vi "sort channels.vi"(7 "Type":T3=enum."Input Register", 8 "error in (no error)":errorcluster, 9 "Starting Index":i32, 10 "Group Name":string, 11 "Item Ref in":T1 format="%.0x") -> (0 "error out":errorcluster, 1 "Next Index":i32, 2 "Inputs":T2[](array[typedef]), 3 "Parent Ref out":T1 format="%.0x", 4 "Refs":T1[](array[typedef]) format="%.0x", 5 "Outputs":T2[](array[typedef]))   [LabVIEW 2015]
uses:
  <vilib>/NI Veristand/Custom Device API/Custom Device API.lvlib
  Modbus Type.ctl
  Shared/Modbus Master Shared.lvlib
  Shared/Controls/Data Model/Channel.ctl
  Modbus Master System Explorer.lvlib
  Shared/Constants.vi
  Shared/Controls/Data Model/DataType.ctl
  Shared/Controls/Data Model/Mapping.ctl
  <vilib>/NI Veristand/Custom Device API/Get Item Property (I32).vi
  <vilib>/NI Veristand/Custom Device API/Custom Device Item Ref.ctl
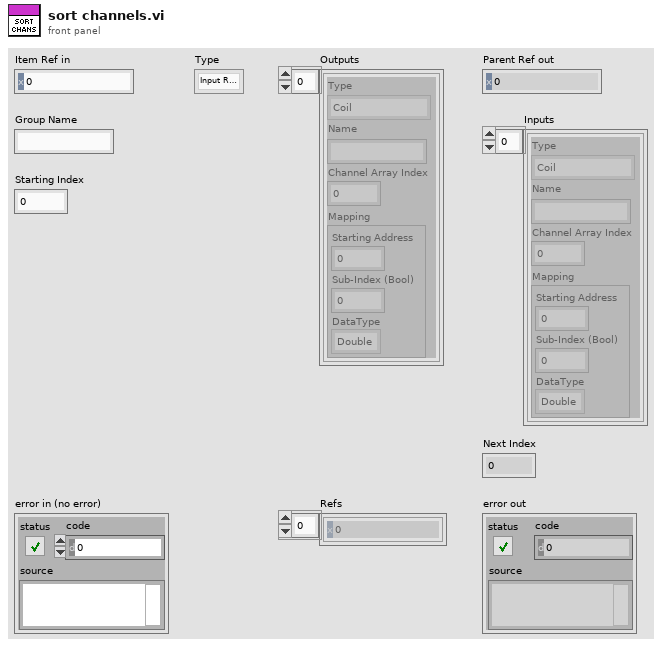
[diagram p1: front panel]
types:
  T1 = typedef "Custom Device API.lvlib/Custom Device Item Ref.ctl" = u64
  T2 = typedef "Modbus Master Shared.lvlib/Channel.ctl" = cluster{"Type":T3, "Name":string, "Channel Array Index":i32, "Mapping":T4}
  T3 = typedef "Modbus Master Shared.lvlib/Modbus Type.ctl" = enum16{"Coil", "Discrete Input", "Holding Register", "Input Register"}
  T4 = typedef "Modbus Master Shared.lvlib/Mapping.ctl" = cluster{"Starting Address":u16, "Sub-Index (Bool)":u16, "DataType":T5}
  T5 = typedef "Modbus Master Shared.lvlib/DataType.ctl" = enum16{"Double", "Single", "I64", "I32", "I16", "I8", "U64", "U32", "U16", "U8", "Boolean", "String"}
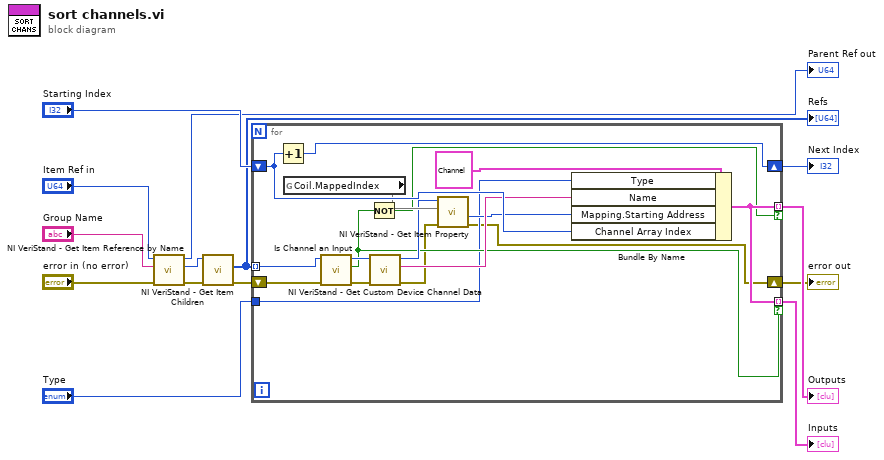
[diagram p0: block diagram]
diagram:
  n1 = call <vilib>:"NI VeriStand - Get Item Reference by Name.vi"("error in (no error)"="error in (no error)", "Item Name"="Group Name", "Parent Ref in"="Item Ref in") -> ("error out"=w4:errorcluster, "Item Ref"=w8:T1, "Parent Ref out"=→"Parent Ref out":T1)  [unwired: 5 in, 1 out]
  n2 = call <vilib>:"NI VeriStand - Get Item Children.vi"("error in (no error)"=w4, "Item Ref in"=w8) -> ("error out"=w2:errorcluster, "Child Refs"=w9:T1[])  [unwired: 6 in, 2 out]
  "Refs" <- w9
  n3 = for {
    tunnel: w9 -> [w31] mode=indexing
    shift-right: [w28] -> w12
    shift-left: "Starting Index" -> [w29]
    tunnel: [w22] -> w13 mode=indexing if=w21
    tunnel: [w22] -> w14 mode=indexing if=w15
    tunnel: "Type" -> [w20]
    shift-right: [w16] -> w1
    shift-left: w2 -> [w19]
    n4 = Increment(x=w29) -> (x+1=w28:i32)
    n5 = global read "Constants.vi" "Coil.MappedIndex"() -> (w25)
    n6 = call "Is Channel an Input"("error in (no error)"=w19, "Item Ref in"=w31) -> ("error out"=w18:errorcluster, "input?"=w21:bool, "Channel Ref out"=w30:T1)  [unwired: 7 in]
    n7 = Not(x=w21) -> (.not. x?=w15:bool)
    n8 = call <vilib>:"NI VeriStand - Get Custom Device Channel Data.vi"("error in (no error)"=w18, "Channel Ref in"=w30) -> ("error out"=w17:errorcluster, "Channel Name"=w26:string, "Channel Ref out"=w24:T1)  [unwired: 4 in, 3 out]
    n9 = call-poly <vilib>:"NI VeriStand - Get Item Property.vi"("error in (no error)"=w17, "Property Name"=w25, "Item Ref in"=w24) -> ("error out"=w16:errorcluster, "Value"=w23:i32)  [unwired: 5 in, 2 out]
    n10 = Bundle By Name(cluster=T2 {"Type"=enum."Coil", "Name"="", "Channel Array Index"=0, "Mapping"={"Starting Address"=0, "Sub-Index (Bool)"=0, "DataType"=enum."Double"}} ("Channel"), "Type"=w20, "Name"=w26, "Mapping.Starting Address"=w23, "Channel Array Index"=w29) -> (w22:T2)
  }
  "Outputs" <- w14
  "Inputs" <- w13
  "Next Index" <- w12
  "error out" <- w1
